vi "getName.vi"(8 "error in (no error)":errorcluster, 11 "DDSOutput in":refnum<class "DDSOutput.lvclass">) -> (0 "error out":errorcluster, 2 "name":string, 3 "DDSOutput out":refnum<class "DDSOutput.lvclass">)   [LabVIEW 2011, in "Hardware.lvlib" / "Channels.lvlib" / "DDSOutput.lvclass"]
uses:
  DDSOutput.lvclass
  DDSOutput.lvclass/DDSOutput.ctl
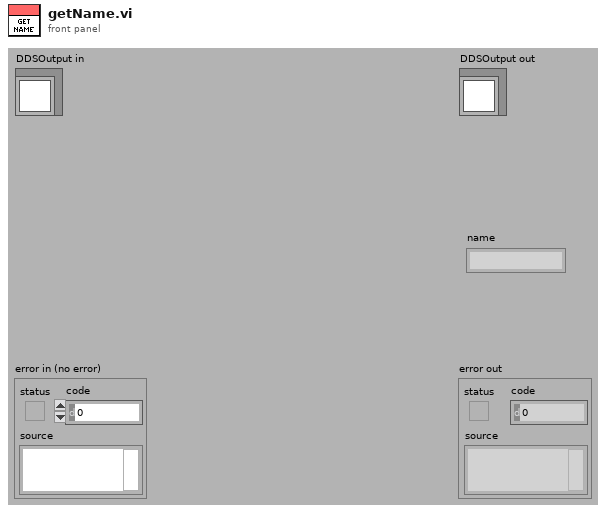
[diagram p1: front panel]
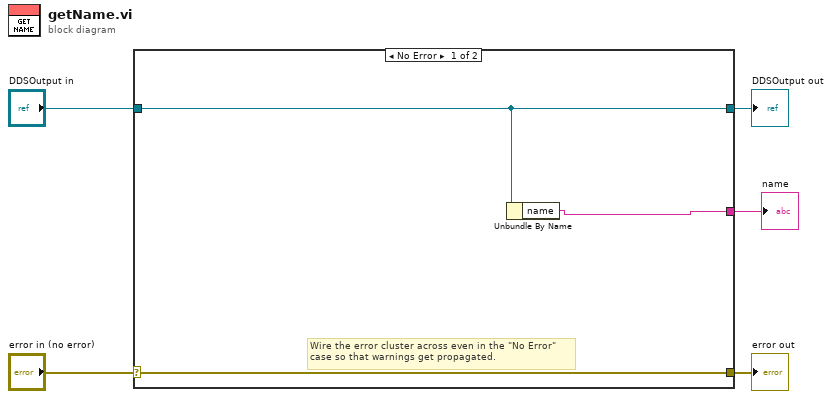
[diagram p0: block diagram]
diagram:
  n1 = case shown="No Error" "error in (no error)" {
    selector: "error in (no error)" -> [w8 w10]
    tunnel: [w8 w10] -> w4
    tunnel: [w7 w9] -> w2
    tunnel: "DDSOutput in" -> [w7 w9]
    tunnel: [w6 _] -> w1
    frame No Error {
      # "Wire the error cluster across even in the \"No Error\"\ncase so that warnings get propagated."
      n2 = Unbundle By Name(w7) -> ("name"=w6:string)
    }
    frame Error {
    }
  }
  "error out" <- w4
  "DDSOutput out" <- w2
  "name" <- w1
